vi "fg_width_padding.vi"(8 "error in (no error)":errorcluster, 11 "width_padding in":u32=10) -> (0 "error out":errorcluster, 3 "width_padding out":u32=10)   [LabVIEW 2015, in "lv-pagination.lvlib"]
doc: "This functional global is used to pad the width of a given cell when re-sizing."
uses:
  lv-pagination.lvlib
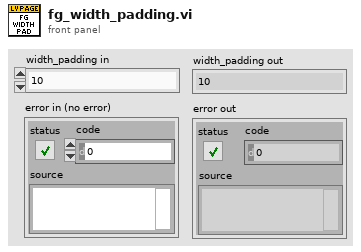
[diagram p1: front panel]
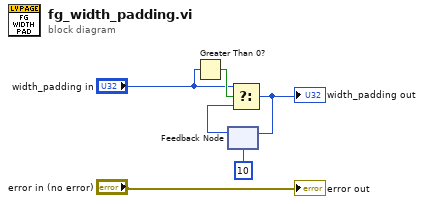
[diagram p0: block diagram]
diagram:
  n1 = Greater Than 0?(x="width_padding in") -> (x > 0?=w2:bool)
  n2 = feedback #1(u32 10 ("x")) -> (w3:u32)
  n3 = Select(t="width_padding in", s=w2, f=w3) -> (s? t:f=w4:u32)
  "width_padding out" <- w4
  n4 = feedback-in #1(w4) -> ()
  "error out" <- "error in (no error)"
